vi "Battery Threshold.vi"(1 "Battery \nThreshold (%)":u8(slide)=5 min=5 max=90 step=5 scale=5.0..90.0) -> (0 "string":string)   [LabVIEW 2026]
panel:
  out "DEC":u8
  out "Boolean array":bool[](array[boolean])
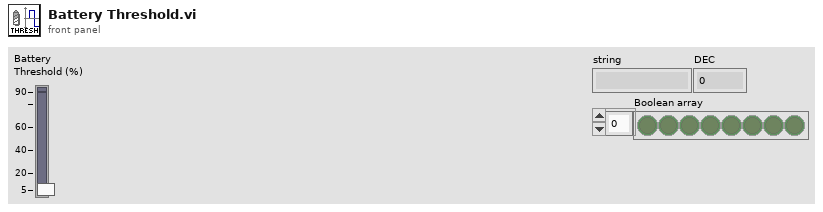
[diagram p1: front panel]
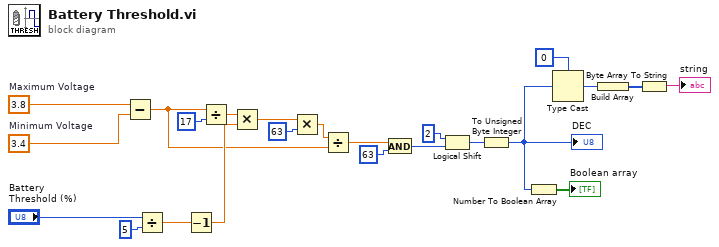
[diagram p0: block diagram]
diagram:
  w16 = 3.4  # Minimum Voltage
  w23 = 3.8  # Maximum Voltage
  n1 = Subtract(x=w23, y=w16) -> (x-y=w13:dbl)
  n2 = Divide(x="Battery \nThreshold (%)", y=u8 5) -> (x/y=w18:dbl)
  n3 = Decrement(x=w18) -> (x-1=w17:dbl)
  n4 = Divide(x=w13, y=17) -> (x/y=w21:dbl)
  n5 = Multiply(x=w21, y=w17) -> (x*y=w11:dbl)
  n6 = Multiply(x=w11, y=u8 63) -> (x*y=w14:dbl)
  n7 = Divide(x=w14, y=w13) -> (x/y=w10:dbl)
  n8 = And(x=w10, y=u8 63) -> (x .and. y?=w8:i32)
  n9 = Logical Shift(y=2 ("x"), x=w8) -> (x << y=w6:i32)
  n10 = To Unsigned Byte Integer(number=w6) -> (unsigned 8bit integer=w3:u8)
  "DEC" <- w3
  n11 = Number To Boolean Array(number=w3) -> (Boolean array=→"Boolean array":bool[])
  n12 = Type Cast(type=u8 0, x=w3) -> (*(type *) &x=w1:u8)
  n13 = Build Array(w1) -> (w4:u8[])
  n14 = Byte Array To String(unsigned byte array=w4) -> (string=→"string":string)
